vi "gyro -- launch async sweeper server.vi"(8 "fitter event pair":T1, 9 "async sweeper event pair":T1, 11 "sweeper server event pair":T1) -> (2 "reference out":refnum<vi>)   [LabVIEW 2018]
uses:
  server talkback message type.ctl
  server talkto message type.ctl
  server talk-to-back pair.ctl
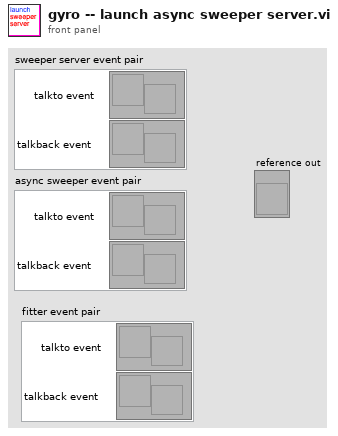
[diagram p1: front panel]
types:
  T1 = typedef "server talk-to-back pair.ctl" = cluster{"talkback event":refnum<user-event>, "talkto event":refnum<user-event>}
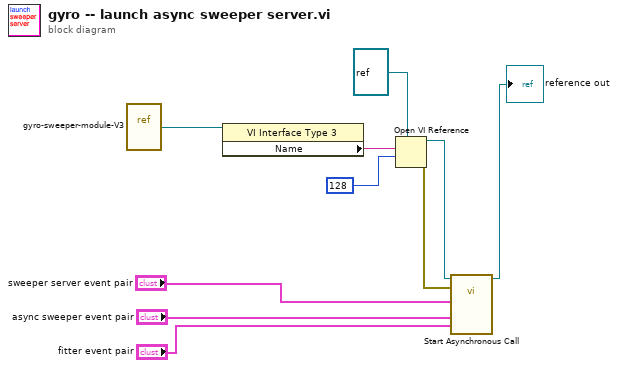
[diagram p0: block diagram]
diagram:
  n1 = vi-ref "gyro-sweeper-module-V3.vi"() -> (w9:refnum<vi>)
  n2 = property class="VI Interface Type 3"(reference=w9) -> ("Name"=w8:string)  [unwired: 1 in, 2 out]
  n3 = Open VI Reference(type specifier VI Refnum (for type only)=refnum<vi> refnum, vi path=w8, options=128) -> (vi reference=w5:refnum<vi>, error out=w4:errorcluster)  [unwired: 3 in]
  n4 = call-by-ref "Start Asynchronous Call"(reference=w5, error in=w4, "fitter event pair"="fitter event pair", "async sweeper event pair"="async sweeper event pair", "this sweeper event pair"="sweeper server event pair") -> (reference out=→"reference out":refnum<vi>)  [unwired: 9 in, 1 out]
